vi "Remove Default Connection.vi"(0 "vi reference":refnum<vi>, 11 "error in":errorcluster) -> (4 "vi reference out":refnum<vi>, 15 "error out":errorcluster)   [LabVIEW 2021, in "Converter.lvlib"]
uses:
  Converter.lvlib
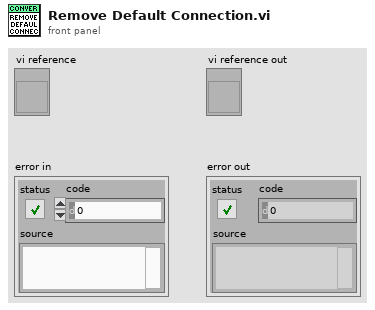
[diagram p1: front panel]
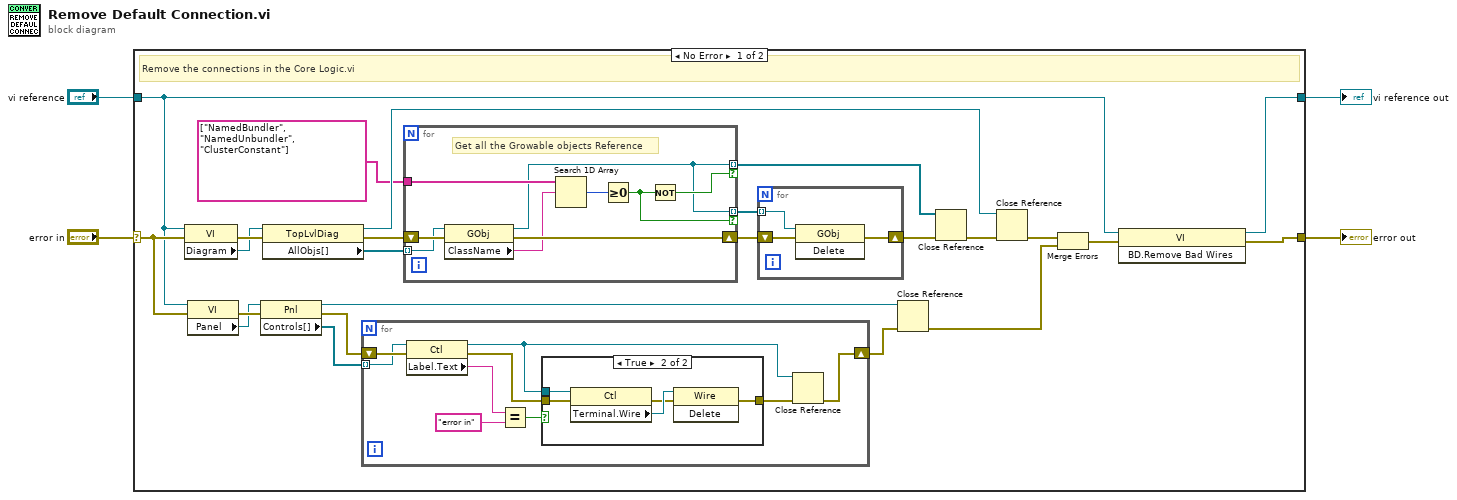
[diagram p0: block diagram]
diagram:
  n1 = case shown="No Error" "error in" {
    selector: "error in" -> [w17 w57]
    tunnel: [w7 w57] -> w1
    tunnel: "vi reference" -> [w5 w56]
    tunnel: [w15 w56] -> w2
    frame No Error {
      # "Remove the connections in the Core Logic.vi"
      n2 = property class="VI"(reference=w5, error in=w17) -> (error out=w28:errorcluster, "Diagram"=w22:refnum<vi>)  [unwired: 1 out]
      n3 = property class="VI"(reference=w5, error in=w17) -> (error out=w20:errorcluster, "Panel"=w14:refnum<vi>)  [unwired: 1 out]
      n4 = property class="Pnl"(reference=w14, error in=w20) -> (reference out=w12:refnum<vi>, error out=w19:errorcluster, "Controls[]"=w21:refnum<vi>[])
      n5 = property class="TopLvlDiag"(reference=w22, error in=w28) -> (reference out=w16:refnum<vi>, error out=w10:errorcluster, "AllObjs[]"=w11:refnum<vi>[])
      n6 = for {
        tunnel: w21 -> [w29] mode=indexing
        shift-right: [w32] -> w13
        shift-left: w19 -> [w35]
        n7 = property class="Ctl"(reference=w29, error in=w35) -> (reference out=w30:refnum<vi>, error out=w34:errorcluster, "Label.Text"=w37:string)
        n8 = Equal?(x=w37, y="error in") -> (x = y?=w36:bool)
        n9 = case shown="True" w36 {
          tunnel: w30 -> [_ w43]
          tunnel: w34 -> [w38 w39]
          tunnel: [w38 w40] -> w33
          frame False {
          }
          frame True {
            n10 = property class="Ctl"(reference=w43, error in=w39) -> (error out=w41:errorcluster, "Terminal.Wire"=w42:refnum<vi>)  [unwired: 1 out]
            n11 = invoke class="Wire" method="Delete"(reference=w42, error in=w41) -> (error out=w40:errorcluster)  [unwired: 1 in, 2 out]
          }
        }
        n12 = Close Reference(reference=w30, error in (no error)=w33) -> (error out=w32:errorcluster)
      }
      n13 = for {
        tunnel: string[] ["NamedBundler", "NamedUnbundler", "ClusterConstant"] -> [w54]
        tunnel: [w49] -> w26 mode=indexing if=w48
        tunnel: [w49] -> w9 mode=indexing if=w50
        shift-right: [w52] -> w25
        shift-left: w10 -> [w53]
        tunnel: w11 -> [w47] mode=indexing
        # "Get all the Growable objects Reference"
        n14 = property class="GObj"(reference=w47, error in=w53) -> (reference out=w49:refnum<vi>, error out=w52:errorcluster, "ClassName"=w51:string)
        n15 = Search 1D Array(1D array=w54, element=w51) -> (index of element=w55:i32)  [unwired: 1 in]
        n16 = Greater Or Equal To 0?(x=w55) -> (x >= 0?=w48:bool)
        n17 = Not(x=w48) -> (.not. x?=w50:bool)
      }
      n18 = for {
        tunnel: w26 -> [w46] mode=indexing
        shift-right: [w44] -> w24
        shift-left: w25 -> [w45]
        n19 = invoke class="GObj" method="Delete"(reference=w46, error in=w45) -> (error out=w44:errorcluster)  [unwired: 1 in, 2 out]
      }
      n20 = Close Reference(reference=w12, error in (no error)=w13) -> (error out=w8:errorcluster)
      n21 = Close Reference(reference=w9, error in (no error)=w24) -> (error out=w27:errorcluster)
      n22 = Close Reference(reference=w16, error in (no error)=w27) -> (error out=w23:errorcluster)
      n23 = Merge Errors(w23, w8) -> (w18:errorcluster)
      n24 = invoke class="VI" method="BD.Remove Bad Wires"(reference=w5, error in=w18) -> (reference out=w15:refnum<vi>, error out=w7:errorcluster)  [unwired: 1 in, 1 out]
    }
    frame Error {
    }
  }
  "error out" <- w1
  "vi reference out" <- w2
